vi "Create Rotation Matrices.vi"(10 "Delta Time in [s]":dbl, 11 "Theta in":dbl) -> (1 "Rotation X Matrix":sgl[][](array[numeric]), 2 "Rotation Z Matrix":sgl[][](array[numeric]), 3 "Theta out":dbl)   [LabVIEW 2020, in "3D.lvlib"]
uses:
  Libraries/3D/3D.lvlib
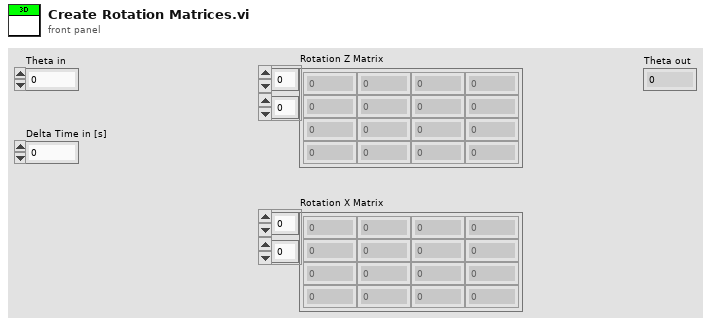
[diagram p1: front panel]
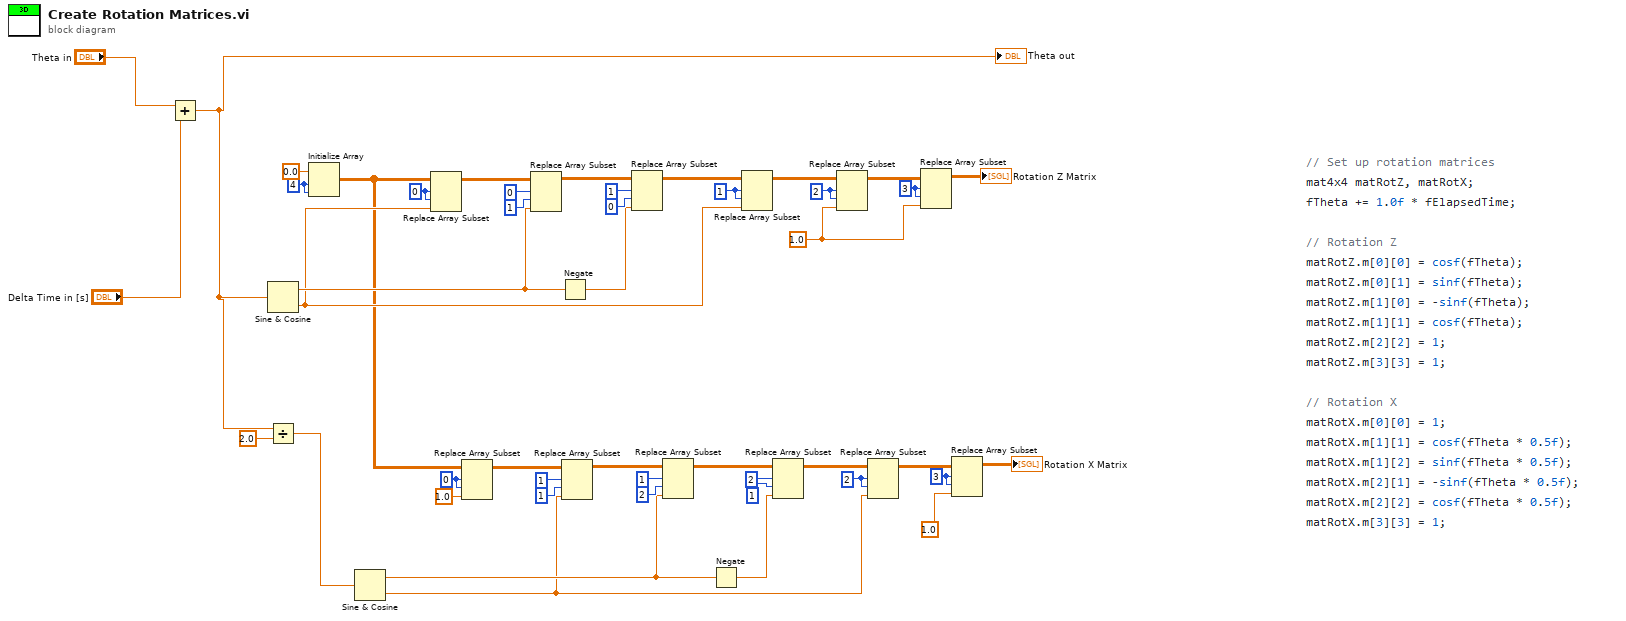
[diagram p0: block diagram]
diagram:
  w24 = 3 ("index (row)")
  w22 = 2 ("index (row)")
  w12 = 0 ("index (row)")
  w31 = sgl 1.0 ("new element/subarray")
  w32 = 3 ("index (row)")
  w34 = 2 ("index (row)")
  w35 = 1 ("index (row)")
  w44 = 0 ("index (row)")
  w45 = 4 ("dimension size")
  n1 = Add(x="Theta in", y="Delta Time in [s]") -> (x+y=w2:dbl)
  "Theta out" <- w2
  n2 = Sine & Cosine(0:w2) -> (1:w30:dbl, 2:w28:dbl)
  n3 = Divide(x=w2, y=2.0) -> (x/y=w9:dbl)
  n4 = Initialize Array(sgl 0.0 ("element"), w45, w45) -> (w11:sgl[][])
  n5 = Sine & Cosine(0:w9) -> (1:w7:dbl, 2:w5:dbl)
  n6 = Replace Array Subset(array=w11, new element=w28, index (row)=w44, index (col)=w44) -> (w43:sgl[][])
  n7 = Replace Array Subset(array=w11, new element=sgl 1.0 ("new element/subarray"), index (row)=w12, index (col)=w12) -> (w13:sgl[][])
  n8 = Replace Array Subset(array=w43, new element=w30, index (row)=0, index (col)=1 ("disabled index (col)")) -> (w40:sgl[][])
  n9 = Negate(x=w30) -> (-x=w29:dbl)
  n10 = Replace Array Subset(array=w13, new element=w5, index (row)=1, index (col)=1 ("disabled index (col)")) -> (w16:sgl[][])
  n11 = Replace Array Subset(array=w40, new element=w29, index (row)=1, index (col)=0 ("index (row)")) -> (w39:sgl[][])
  n12 = Replace Array Subset(array=w16, new element=w7, index (row)=1, index (col)=2 ("index (row)")) -> (w17:sgl[][])
  n13 = Negate(x=w7) -> (-x=w6:dbl)
  n14 = Replace Array Subset(array=w39, new element=w28, index (row)=w35, index (col)=w35) -> (w38:sgl[][])
  n15 = Replace Array Subset(array=w17, new element=w6, index (row)=2, index (col)=1 ("index (row)")) -> (w18:sgl[][])
  n16 = Replace Array Subset(array=w38, new element=w31, index (row)=w34, index (col)=w34) -> (w33:sgl[][])
  n17 = Replace Array Subset(array=w18, new element=w5, index (row)=w22, index (col)=w22) -> (w23:sgl[][])
  n18 = Replace Array Subset(array=w33, new element=w31, index (row)=w32, index (col)=w32) -> (→"Rotation Z Matrix":sgl[][])
  n19 = Replace Array Subset(array=w23, new element=sgl 1.0 ("new element/subarray"), index (row)=w24, index (col)=w24) -> (→"Rotation X Matrix":sgl[][])
